vi "Debug Get Config Settings.vi"() -> ()   [LabVIEW 2021]
uses:
  Ethernet/Ethernet_BS1201.lvclass
panel:
  out "UDP Data Enable":bool=TRUE
  out "UDP Data Port":i32=54321
  out "UDPDataPeriod_mS":i32=5
  in  "UDP port":u16=54321
  in  "TCP port":u16=12345
  in  "Box IP address":string="192.168.1.100"
  out "Configuration Data":string
  out "Received":bool
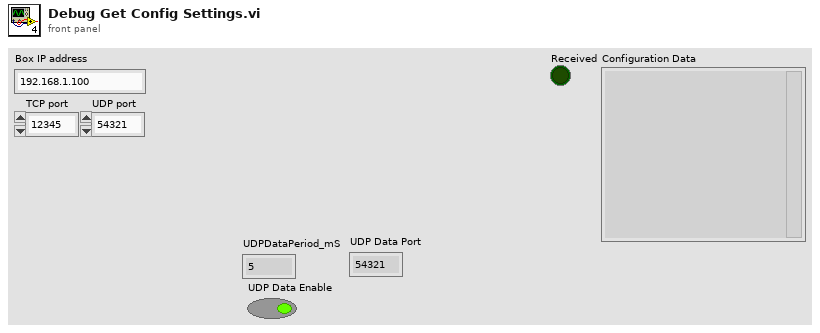
[diagram p1: front panel]
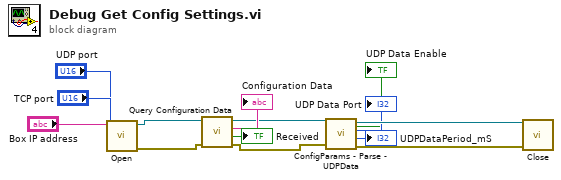
[diagram p0: block diagram]
diagram:
  n1 = call "Open.vi"("UDP port"="UDP port", "TCP port"="TCP port", "Box IP address"="Box IP address") -> ("error out"=w13:errorcluster, "ENET out"=w14:refnum<class "Ethernet_BS1201.lvclass">)  [unwired: 7 in]
  n2 = call-dynamic "Query Configuration Data.vi"("error in (no error)"=w13, "Ethernet in"=w14) -> ("error out"=w5:errorcluster, "Received"=→"Received":bool, "Configuration Data"=→"Configuration Data":string, "Ethernet out"=w7:refnum<class "Ethernet_BS1201.lvclass">)  [unwired: 6 in]
  n3 = call-dynamic "ConfigParams - Parse - UDPData.vi"("error in (no error)"=w5, "Ethernet in"=w7) -> ("error out"=w4:errorcluster, "UDPDataPeriod_mS"=→"UDPDataPeriod_mS":i32, "UDP Data Port"=→"UDP Data Port":i32, "Ethernet out"=w6:refnum<class "Ethernet_BS1201.lvclass">, "UDP Data Enable"=→"UDP Data Enable":bool)  [unwired: 5 in]
  n4 = call-dynamic "Close.vi"("error in (no error)"=w4, "ENET in"=w6) -> ()  [unwired: 9 in, 1 out]
